vi "Test Ramp Field Y.vi"(8 "error in (no error)":errorcluster, 9 "Target Field Rate (T/min)":dbl=0.05 format="%#_13g", 10 "Target Field (T)":dbl=0.05 format="%#_13g", 11 "Instrument.OxfordVRM in":refnum<class "Instrument.OxfordVRM.lvclass">) -> (0 "error out":errorcluster, 3 "Instrument.OxfordVRM out":refnum<class "Instrument.OxfordVRM.lvclass">)   [LabVIEW 2016, in "Instrument.OxfordVRM.lvclass"]
uses:
  Instrument.OxfordVRM.lvclass
  <vilib>/addons/_JKI Toolkits/Caraya/classes/Assert/Assert Not Error.vi
  <vilib>/addons/_JKI Toolkits/Caraya/classes/Assert/Assert Equal Value and Type_Variant.vi
  <vilib>/addons/_JKI Toolkits/Caraya/classes/Assert/Assert Almost Equal_Float.vi
  <vilib>/addons/_JKI Toolkits/Caraya/classes/Test/Test.lvclass
  <vilib>/addons/_JKI Toolkits/Caraya/classes/Assert/Assert.lvclass
panel:
  out "Power Supply Field (T)":dbl
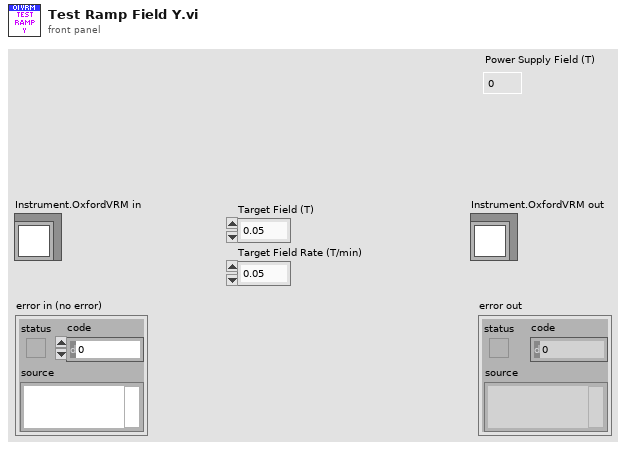
[diagram p1: front panel]
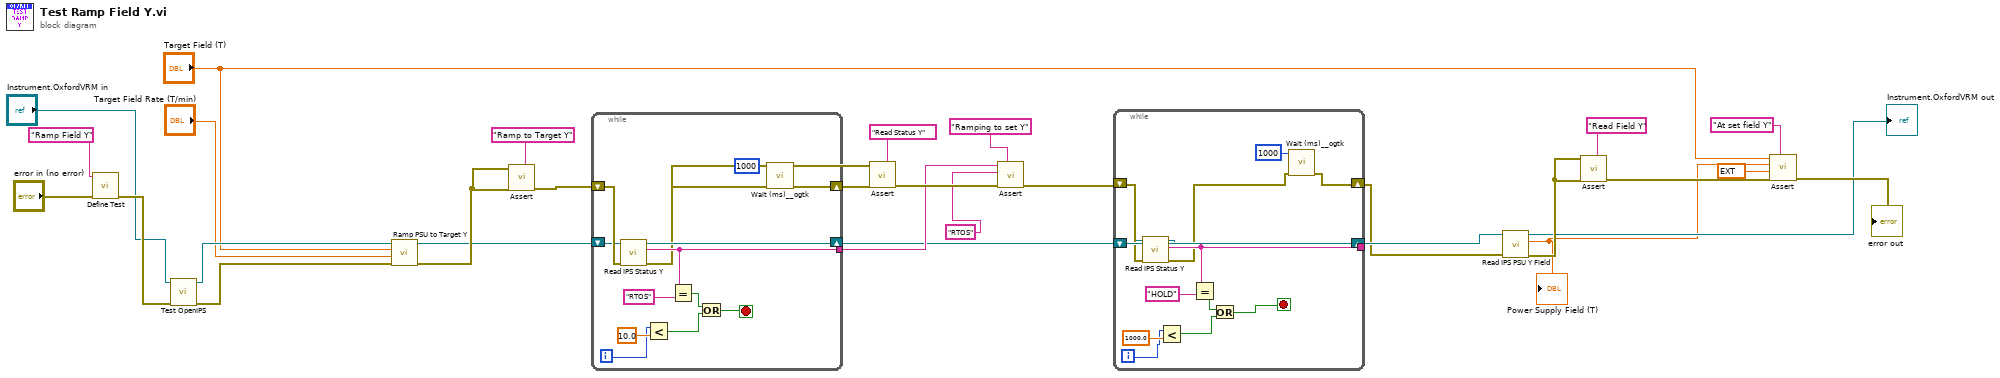
[diagram p0: block diagram]
diagram:
  n1 = call <vilib>:"Define Test.vi"("error in (no error)"="error in (no error)", "Label (VI Title)"="Ramp Field Y") -> ("error out"=w10:errorcluster)  [unwired: 9 in]
  n2 = call "Test OpenIPS.vi"("error in (no error)"=w10, "Instrument.OxfordVRM in"="Instrument.OxfordVRM in") -> ("error out"=w3:errorcluster, "Instrument.OxfordVRM out"=w4:refnum<class "Instrument.OxfordVRM.lvclass">)  [unwired: 8 in]
  n3 = call "Ramp PSU to Target Y.vi"("error in (no error)"=w3, "Target Rate (T/min)"="Target Field Rate (T/min)", "Target Field (T)"="Target Field (T)", "Instrument.OxfordVRM in"=w4) -> ("error out"=w23:errorcluster, "Instrument.OxfordVRM out"=w21:refnum<class "Instrument.OxfordVRM.lvclass">)  [unwired: 6 in]
  n4 = call-poly <vilib>:"Assert.vi"("Label"="Ramp to Target Y", "error in (no error)"=w23, "Not Error?"=w23) -> ("error out"=w22:errorcluster)  [unwired: 8 in]
  n5 = while {
    tunnel: [w39] -> w17
    shift-right: [w35] -> w19
    shift-left: w22 -> [w42]
    shift-right: [w40] -> w15
    shift-left: w21 -> [w41]
    i -> [w33]
    stop <- w32 stop-if-true
    n6 = call "Read IPS Status Y.vi"("error in (no error)"=w42, "Instrument.OxfordVRM in"=w41) -> ("error out"=w36:errorcluster, "Status"=w39:string, "Instrument.OxfordVRM out"=w40:refnum<class "Instrument.OxfordVRM.lvclass">)  [unwired: 7 in]
    n7 = Less?(x=w33, y=10.0) -> (x < y?=w30:bool)
    n8 = Equal?(x=w39, y="RTOS") -> (x = y?=w31:bool)
    n9 = Or(x=w31, y=w30) -> (x .or. y?=w32:bool)
    n10 = call <userlib>:"Wait (ms)__ogtk.vi"("error in (no error)"=w36, "milliseconds to wait"=u32 1000) -> ("error out"=w35:errorcluster)  [unwired: 8 in, 1 out]
  }
  n11 = call-poly <vilib>:"Assert.vi"("Label"="Read Status Y", "error in (no error)"=w19, "Not Error?"=w19) -> ("error out"=w18:errorcluster)  [unwired: 8 in]
  n12 = call-poly <vilib>:"Assert.vi"("Label"="Ramping to set Y", "error in (no error)"=w18, "Y"="RTOS", "X"=w17) -> ("error out"=w6:errorcluster)  [unwired: 7 in]
  n13 = while {
    tunnel: [w52] -> _
    shift-right: [w48] -> w5
    shift-left: w6 -> [w55]
    shift-right: [w53] -> _
    shift-left: _ -> [w54]
    i -> [w43]
    stop <- w44 stop-if-true
    n14 = call "Read IPS Status Y.vi"("error in (no error)"=w55, "Instrument.OxfordVRM in"=w54) -> ("error out"=w49:errorcluster, "Status"=w52:string, "Instrument.OxfordVRM out"=w53:refnum<class "Instrument.OxfordVRM.lvclass">)  [unwired: 7 in]
    n15 = Less?(x=w43, y=1000.0) -> (x < y?=w46:bool)
    n16 = Equal?(x=w52, y="HOLD") -> (x = y?=w45:bool)
    n17 = Or(x=w45, y=w46) -> (x .or. y?=w44:bool)
    n18 = call <userlib>:"Wait (ms)__ogtk.vi"("error in (no error)"=w49, "milliseconds to wait"=u32 1000) -> ("error out"=w48:errorcluster)  [unwired: 8 in, 1 out]
  }
  n19 = call "Read IPS PSU Y Field.vi"("error in (no error)"=w5, "Instrument.OxfordVRM in"=w15) -> ("error out"=w13:errorcluster, "Power Supply Field (T)"=w8:dbl, "Instrument.OxfordVRM out"=→"Instrument.OxfordVRM out":refnum<class "Instrument.OxfordVRM.lvclass">)  [unwired: 7 in]
  "Power Supply Field (T)" <- w8
  n20 = call-poly <vilib>:"Assert.vi"("Label"="Read Field Y", "error in (no error)"=w13, "Not Error?"=w13) -> ("error out"=w12:errorcluster)  [unwired: 8 in]
  n21 = call-poly <vilib>:"Assert.vi"("Label"="At set field Y", "error in (no error)"=w12, "Tolerance"=ext 0.00099999999999999999996, "Y"=w8, "X"="Target Field (T)") -> ("error out"=→"error out":errorcluster)  [unwired: 6 in]
